vi "LidarRead.vi"(1 "LidarDevRef":T1={"DevStatus"={"status"=FALSE, "code"=0, "source"=""}, "Controller"=enum."Controller 1", "Device Address"=0, "Handle"=0, "I2C Bus"=enum."Invalid"} {"Device Address" format="%.0x"}) -> (0 "Distance(cm)":u16)   [LabVIEW 2014]
uses:
  <vilib>/Rock Robotics/WPI/I2C/WPI_I2CDevRef.ctl
  <vilib>/Rock Robotics/SystemInterfaces/Typedef/FPGA_TypedefDigitalModule.ctl
  <vilib>/Rock Robotics/SystemInterfaces/i2clib/i2c_bus.ctl
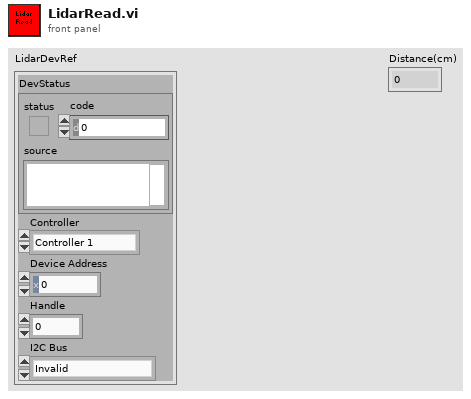
[diagram p1: front panel]
types:
  T1 = typedef "WPI_I2CDevRef.ctl" = cluster{"DevStatus":errorcluster, "Controller":T2, "Device Address":u8, "Handle":i32, "I2C Bus":T3}
  T2 = typedef "FPGA_TypedefDigitalModule.ctl" = enum16{"Controller 1"}
  T3 = typedef "i2c_bus.ctl" = enum16{"I2C On-Board", "I2C MXP", "Invalid"}
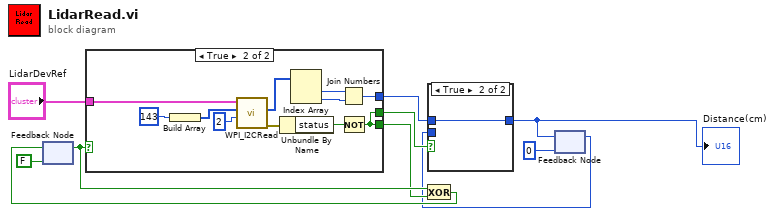
[diagram p0: block diagram]
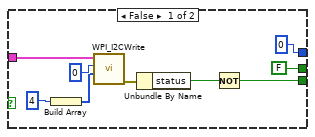
[diagram p3: hidden frame]
diagram:
  n1 = feedback #1(FALSE) -> (w8:bool)
  n2 = case shown="True" w8 {
    tunnel: "LidarDevRef" -> [w19 w30]
    tunnel: [w14 w24] -> w6
    tunnel: [FALSE w24] -> w5
    tunnel: [u16 0 w20] -> w4
    frame False {
      n3 = Build Array(u8 4) -> (w16:u8[])
      n4 = call <vilib>:"WPI_I2CWrite.vi"("I2CDataToSend"=w16, "I2CRegister"=u8 0, "I2CDevRef"=w19) -> ("error out"=w15:errorcluster)  [unwired: 7 in, 1 out]
      n5 = Unbundle By Name(w15) -> ("status"=w13:bool)
      n6 = Not(x=w13) -> (.not. x?=w14:bool)
    }
    frame True {
      n7 = Build Array(u8 143) -> (w28:u8[])
      n8 = call <vilib>:"WPI_I2CRead.vi"("I2CBytesToRead"=u8 2, "I2CRegister"=w28, "I2CDevRef"=w30) -> ("error out"=w26:errorcluster, "Data Out"=w23:u8[])  [unwired: 6 in, 1 out]
      n9 = Unbundle By Name(w26) -> ("status"=w25:bool)
      n10 = Index Array(array=w23) -> (element #1=w22:u8, element #2=w21:u8)  [unwired: 2 in]
      n11 = Join Numbers(hi=w22, lo=w21) -> ((hi.lo)=w20:u16)
      n12 = Not(x=w25) -> (.not. x?=w24:bool)
    }
  }
  n13 = Exclusive Or(1:w6, 2:w8) -> (0:w10:bool)
  n14 = feedback-in #1(w10) -> ()
  n15 = feedback #2(u16 0) -> (w2:u16)
  n16 = case shown="True" w5 {
    tunnel: w4 -> [_ w32]
    tunnel: [w31 w32] -> w1
    tunnel: w2 -> [w31 _]
    frame False {
    }
    frame True {
    }
  }
  "Distance(cm)" <- w1
  n17 = feedback-in #2(w1) -> ()
